vi "Moisture SASS.vi"() -> ()   [LabVIEW 2013]
uses:
  <vilib>/myRIO/Instrument Drivers/Onboard IO/AI/vis/Smart Open.vi
  <vilib>/myRIO/Instrument Drivers/Onboard IO/AI/vis/Read.vi
  <vilib>/myRIO/Instrument Drivers/Onboard IO/AI/vis/Open.vi
  <vilib>/Utility/error.llb/Error Cluster From Error Code.vi
panel:
  out "MOISTURE LEVEL(ppm)":dbl
  # "AJAY KUMAR GARG ENGINEERING COLLEGE\n                 NI-YANTRA 2017\n                      NIY-135"
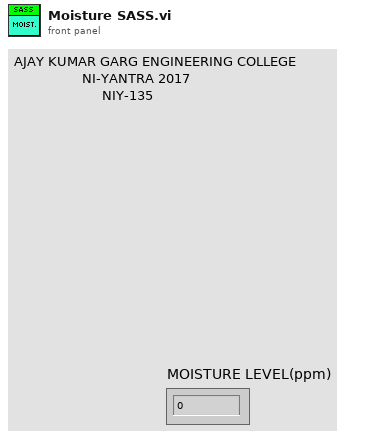
[diagram p1: front panel]
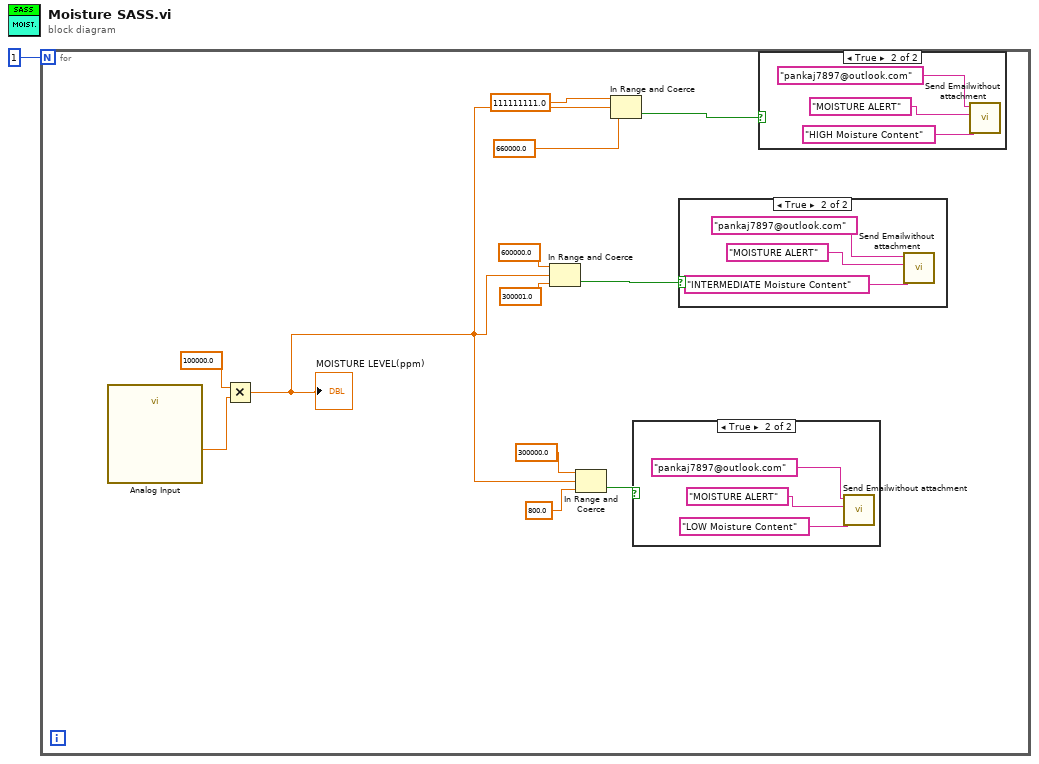
[diagram p0: block diagram]
diagram:
  n1 = for {
    N: 1 -> [_]
    n2 = call "Analog Input"() -> ("A/AI0 (Pin 3)"=w13:dbl)  [unwired: 26 in, 1 out]
    n3 = Multiply(x=100000.0, y=w13) -> (x*y=w2:dbl)
    "MOISTURE LEVEL(ppm)" <- w2
    n4 = In Range and Coerce(upper limit=600000.0, x=w2, lower limit=300001.0 ("upper limit")) -> (In Range?=w9:bool)  [unwired: 1 out]
    n5 = In Range and Coerce(upper limit=300000.0, x=w2, lower limit=800.0 ("upper limit")) -> (In Range?=w4:bool)  [unwired: 1 out]
    n6 = In Range and Coerce(upper limit=111111111.0, x=w2, lower limit=660000.0 ("upper limit")) -> (In Range?=w3:bool)  [unwired: 1 out]
    n7 = case shown="True" w4 {
      frame False {
      }
      frame True {
        n8 = call "Send Emailwithout attachment.vi"("To: 2"="pankaj7897@outlook.com", "Subject 2"="MOISTURE ALERT", "Message 2"="LOW Moisture Content") -> ()  [unwired: 8 in]
      }
    }
    n9 = case shown="True" w9 {
      frame False {
      }
      frame True {
        n10 = call "Send Emailwithout attachment.vi"("To: 2"="pankaj7897@outlook.com", "Subject 2"="MOISTURE ALERT", "Message 2"="INTERMEDIATE Moisture Content") -> ()  [unwired: 8 in]
      }
    }
    n11 = case shown="True" w3 {
      frame False {
      }
      frame True {
        n12 = call "Send Emailwithout attachment.vi"("To: 2"="pankaj7897@outlook.com", "Subject 2"="MOISTURE ALERT", "Message 2"="HIGH Moisture Content") -> ()  [unwired: 8 in]
      }
    }
  }
